vi "Read Valve Status.vi"(8 "Error In":errorcluster, 10 "Channel (-1:Main)":i32=-1, 11 "VISA resource name":refnum<visa-resource-name>) -> (0 "Error Out":errorcluster, 3 "dup VISA resource name":refnum<visa-resource-name>)   [LabVIEW 2011, in "MGC647C.lvlib"]
doc: "Switch valve of a channel."
uses:
  <instrlib>/MGC647C/MGC647C.lvlib
panel:
  out "Open/close":bool=TRUE
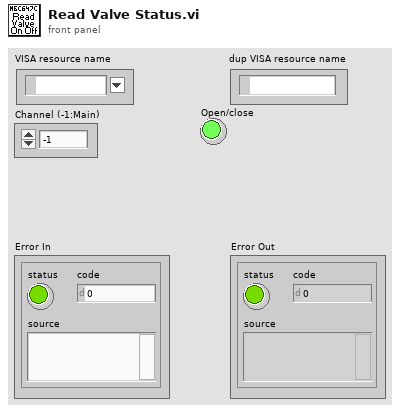
[diagram p1: front panel]
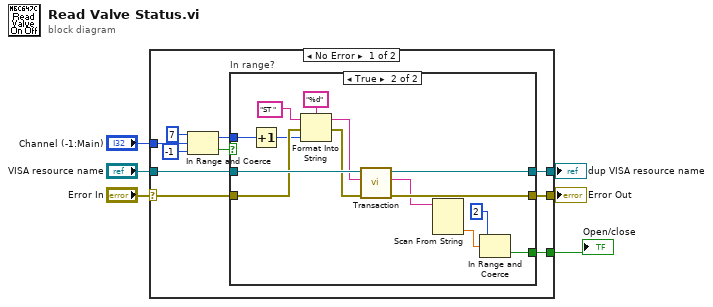
[diagram p0: block diagram]
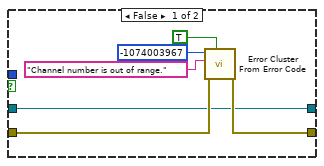
[diagram p2: hidden frame]
diagram:
  n1 = case shown="No Error" "Error In" {
    selector: "Error In" -> [w13 w38]
    tunnel: "VISA resource name" -> [w16 w37]
    tunnel: [w15 w37] -> w5
    tunnel: [w14 w38] -> w4
    tunnel: "Channel (-1:Main)" -> [w10 _]
    tunnel: [w7 _] -> w1
    frame No Error {
      n2 = In Range and Coerce(upper limit=7, x=w10, lower limit=-1) -> (coerced(x)=w9:i32, In Range?=w8:bool)
      n3 = case "In range?" shown="True" w8 {
        tunnel: w16 -> [w20 w36]
        tunnel: [w20 w35] -> w15
        tunnel: [w21 w28] -> w14
        tunnel: w13 -> [w22 w34]
        tunnel: w9 -> [_ w32]
        tunnel: [_ w23] -> w7
        frame False {
          n4 = call <vilib>:"Error Cluster From Error Code.vi"("show call chain? (False)"=TRUE, "error in (no error)"=w22, "error message (\"\")"="Channel number is out of range." ("error message (\"\")"), "error code (0)"=-1074003967) -> ("error out"=w21:errorcluster)  [unwired: 5 in]
        }
        frame True {
          n5 = Increment(x=w32) -> (x+1=w31:i32)
          n6 = Format Into String(format string="%d", initial string="ST " ("string (\"\")"), error in=w34, w31) -> (resulting string=w30:string, error out=w33:errorcluster)
          n7 = call <instrlib>:"Transaction.vi"("Error In"=w33, "Command"=w30, "VISA resource name"=w36) -> ("Error Out"=w28:errorcluster, "Response"=w26:string, "dup VISA resource name"=w35:refnum<visa-resource-name>)  [unwired: 6 in]
          n8 = Scan From String(input string=w26) -> (output 1=w25:dbl)  [unwired: 4 in, 3 out]
          n9 = In Range and Coerce(upper limit=2, x=w25) -> (In Range?=w23:bool)  [unwired: 1 in, 1 out]
        }
      }
    }
    frame Error {
    }
  }
  "dup VISA resource name" <- w5
  "Error Out" <- w4
  "Open/close" <- w1
